vi "setScope.vi"(8 "error in (no error)":errorcluster, 10 "Scope":refnum<class "tBSONDocument.lvclass">, 11 "tBSONJavaScriptWithScope in":refnum<class "tBSONJavaScriptWithScope.lvclass">) -> (0 "error out":errorcluster, 3 "tBSONJavaScriptWithScope out":refnum<class "tBSONJavaScriptWithScope.lvclass">)   [LabVIEW 2013, in "BSON.lvlib" / "tBSONJavaScriptWithScope.lvclass"]
uses:
  tBSONJavaScriptWithScope.lvclass
  tBSONDocument/tBSONDocument.lvclass
  tBSONJavaScriptWithScope.lvclass/tBSONJavaScriptWithScope.ctl
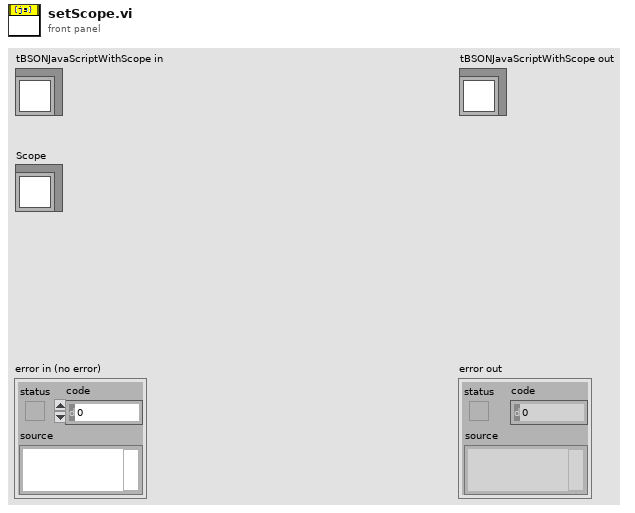
[diagram p1: front panel]
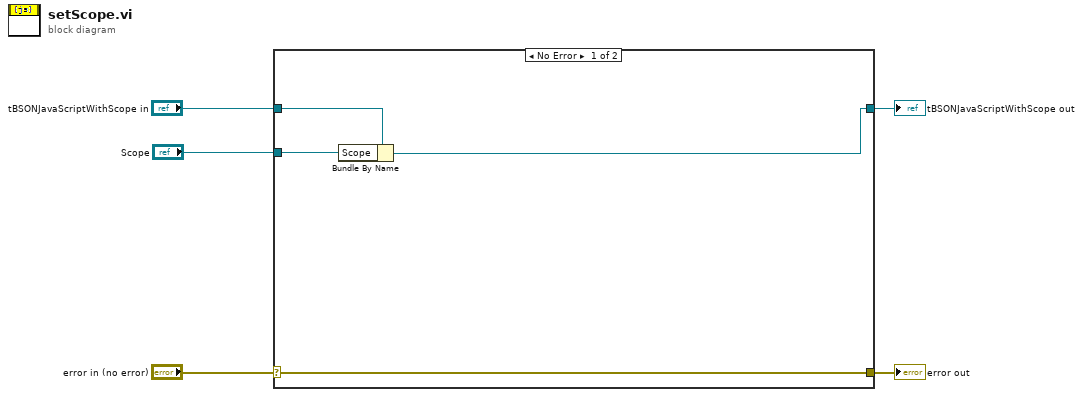
[diagram p0: block diagram]
diagram:
  n1 = case shown="No Error" "error in (no error)" {
    selector: "error in (no error)" -> [w9 w11]
    tunnel: [w9 w11] -> w4
    tunnel: [w6 w10] -> w2
    tunnel: "tBSONJavaScriptWithScope in" -> [w7 w10]
    tunnel: "Scope" -> [w8 _]
    frame No Error {
      n2 = Bundle By Name(cluster=w7, "Scope"=w8) -> (w6:refnum<class "tBSONJavaScriptWithScope.lvclass">)
    }
    frame Error {
    }
  }
  "error out" <- w4
  "tBSONJavaScriptWithScope out" <- w2
